vi "PixyAverageY.vi"(10 "Input":dbl, 11 "Past array Width":dbl[](array[numeric])) -> (2 "Array":dbl[](array[numeric]), 3 "mean":dbl)   [LabVIEW 2016]
uses:
  <vilib>/Analysis/baseanly.llb/Mean (DBL).vi
  <vilib>/Analysis/NI_AALBase.lvlib
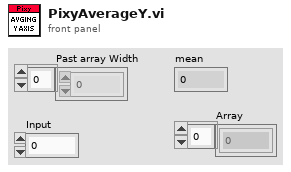
[diagram p1: front panel]
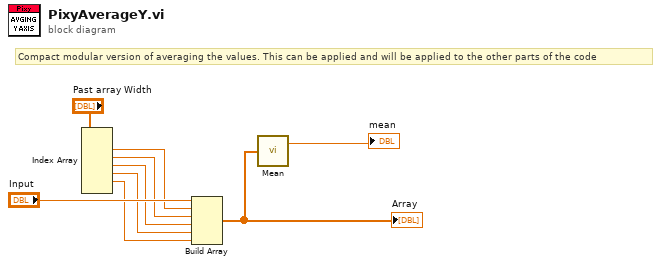
[diagram p0: block diagram]
diagram:
  # "Compact modular version of averaging the values. This can be applied and will be applied to the other parts of the code"
  n1 = Index Array(array="Past array Width") -> (element #1=w5:dbl, element #2=w6:dbl, element #3=w3:dbl, element #4=w2:dbl, element #5=w1:dbl)  [unwired: 6 in, 1 out]
  n2 = Build Array("Input", w5, w6, w3, w2, w1) -> (w9:dbl[])
  "Array" <- w9
  n3 = call-poly <vilib>:"Mean.vi"("X"=w9) -> ("mean"=→"mean":dbl)  [unwired: 1 out]
